vi "RW_turnon-off.vi"(3 "error in (no error)":errorcluster caption="Error IN", 4 "On/Off":bool, 5 "VISAsession":refnum<visa-resource-name>="wavefactoryU5") -> (0 "error out":errorcluster caption="Error OUT", 2 "CopyVISAsession":refnum<visa-resource-name>="wavefactoryU5")   [LabVIEW 2018]
panel:
  out "Elapsed Time":dbl=0.012954899999385816
  # "Have to manually set each Wavefactory \nto 2-phase, sweep, 50 ohms (both channels),\noffsets, sine waves...ugh"
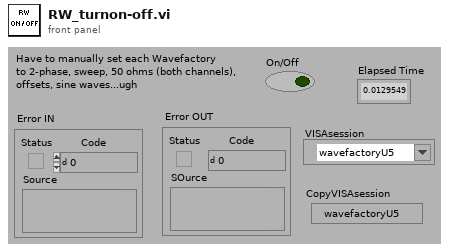
[diagram p1: front panel]
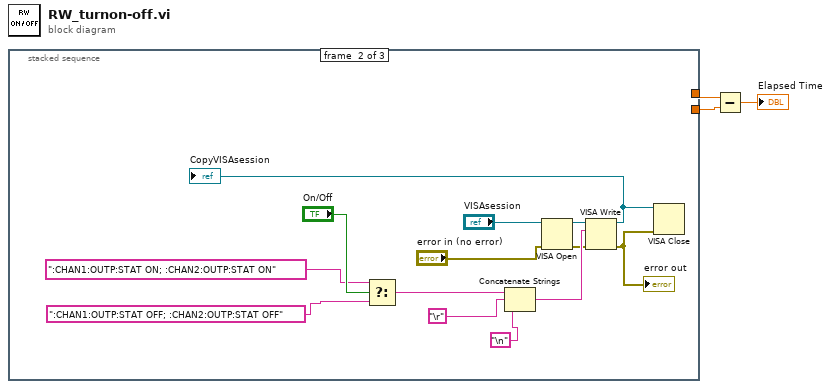
[diagram p0: block diagram]
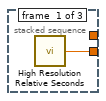
[diagram p2: hidden frame]
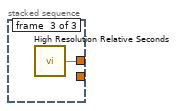
[diagram p3: hidden frame]
diagram:
  n1 = stacked-sequence {
    tunnel: [w4 _ _] -> w2
    tunnel: [_ _ w18] -> w3
    frame #0 {
      n2 = call <vilib>:"High Resolution Relative Seconds.vi"() -> ("relative seconds"=w4:dbl)
    }
    frame #1 {
      n3 = Select(t=":CHAN1:OUTP:STAT ON; :CHAN2:OUTP:STAT ON", s="On/Off", f=":CHAN1:OUTP:STAT OFF; :CHAN2:OUTP:STAT OFF") -> (s? t:f=w9:string)
      n4 = Concatenate Strings(w9, "\r", "\n") -> (w15:string)
      n5 = VISA Open(error in (no error)="error in (no error)", VISA resource name="VISAsession") -> (VISA resource name=w13:refnum<visa-resource-name>, error out=w14:errorcluster)  [unwired: 3 in]
      n6 = VISA Write(VISA resource name=w13, write buffer=w15, error in (no error)=w14) -> (VISA resource name out=w12:refnum<visa-resource-name>, error out=w11:errorcluster)  [unwired: 1 out]
      "error out" <- w11
      "CopyVISAsession" <- w12
      n7 = VISA Close(VISA resource name=w12, error in (no error)=w11) -> ()  [unwired: 1 out]
    }
    frame #2 {
      n8 = call <vilib>:"High Resolution Relative Seconds.vi"() -> ("relative seconds"=w18:dbl)
    }
  }
  n9 = Subtract(x=w3, y=w2) -> (x-y=→"Elapsed Time":dbl)
